vi "NI VeriStand - Get Custom Device Dependencies.vi"(8 "error in (no error)":errorcluster, 11 "Device Ref in":T5 format="%.0x") -> (0 "error out":errorcluster, 2 "Dependencies":T1[](array[typedef]), 3 "Device Ref out":T5 format="%.0x")   [LabVIEW 2020, in "Custom Device Offline API.lvlib"]
uses:
  <vilib>/NI VeriStand/Custom Device Offline API/Custom Device Offline API.lvlib
  <vilib>/NI VeriStand/Custom Device API/Custom Device Item Ref.ctl
  <vilib>/NI VeriStand/Custom Device API/Custom Device File Dependency.ctl
  <vilib>/NI VeriStand/Custom Device API/Path Specification.ctl
  <vilib>/NI VeriStand/Custom Device API/Path Type.ctl
  <vilib>/NI VeriStand/Custom Device API/Custom Device Supported Target.ctl
  NationalInstruments.VeriStand.SystemDefinitionAPI
  <vilib>/NI VeriStand/Custom Device API/Custom Device API.lvlib
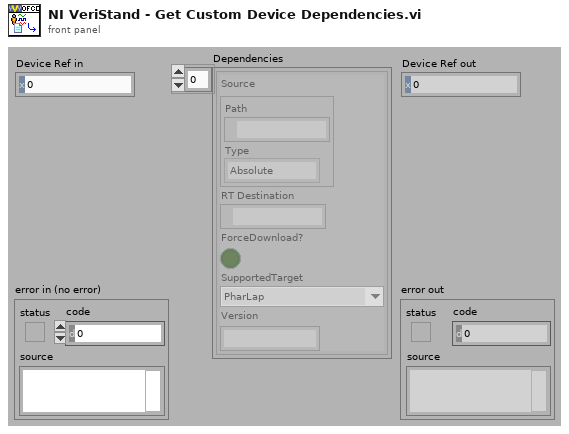
[diagram p1: front panel]
types:
  T1 = typedef "Custom Device API.lvlib/Custom Device File Dependency.ctl" = cluster{"Source":T2, "RT Destination":path, "ForceDownload?":bool, "SupportedTarget":T4, "Version":string}
  T2 = typedef "Custom Device API.lvlib/Path Specification.ctl" = cluster{"Path":path, "Type":T3}
  T3 = typedef "Custom Device API.lvlib/Path Type.ctl" = enum16{"Absolute", "To Base", "To Common Data Dir", "To Application Data Dir"}
  T4 = typedef "Custom Device API.lvlib/Custom Device Supported Target.ctl" = enum16{"All", "PharLap", "VxWorks", "Windows", "Linux_32_ARM", "Linux_x64", "PharLap & Windows", "PharLap & VxWorks", "VxWorks & Windows"}
  T5 = typedef "Custom Device API.lvlib/Custom Device Item Ref.ctl" = u64
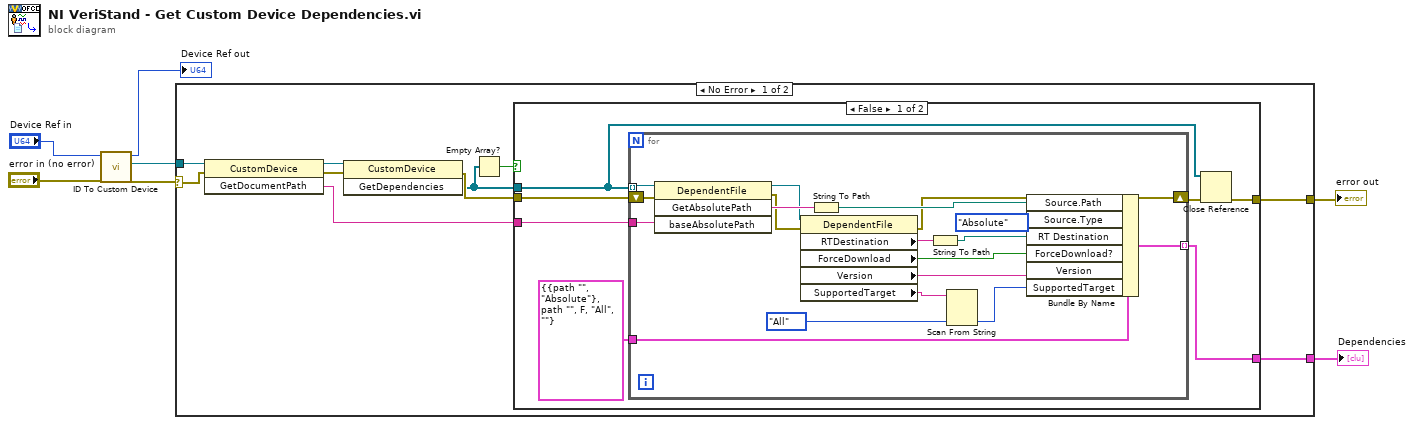
[diagram p0: block diagram]
diagram:
  n1 = call <vilib>:"ID To Custom Device.vi"("error in (no error)"="error in (no error)", "ID in"="Device Ref in") -> ("error out"=w4:errorcluster, "Device"=w3:refnum<k24>, "ID out"=→"Device Ref out":u64)  [unwired: 7 in]
  n2 = case shown="No Error" w4 {
    selector: w4 -> [w16 w44]
    tunnel: w3 -> [w17 _]
    tunnel: [w9 _] -> w2
    tunnel: [w8 w44] -> w1
    frame No Error {
      n3 = invoke class="CustomDevice" method="GetDocumentPath"(reference=w17, error in=w16) -> (reference out=w15:refnum<k24>, error out=w14:errorcluster, "GetDocumentPath"=w12:string)  [unwired: 1 in]
      n4 = invoke class="CustomDevice" method="GetDependencies"(reference=w15, error in=w14) -> (error out=w13:errorcluster, "GetDependencies"=w11:refnum<k24>[])  [unwired: 1 in, 1 out]
      n5 = Empty Array?(array=w11) -> (empty?=w10:bool)
      n6 = case shown="False" w10 {
        tunnel: w13 -> [w23 w43]
        tunnel: w12 -> [w22 _]
        tunnel: w11 -> [w20 _]
        tunnel: [w19 _] -> w9
        tunnel: [w18 w43] -> w8
        frame False {
          n7 = for {
            tunnel: w20 -> [w41] mode=indexing
            tunnel: T1 {"Source"={"Path"=path "", "Type"=enum."Absolute"}, "RT Destination"=path "", "ForceDownload?"=FALSE, "SupportedTarget"=enum."All", "Version"=""} ("Dependency") -> [w42]
            shift-right: [w26] -> w21
            shift-left: w23 -> [w40]
            tunnel: w22 -> [w39]
            tunnel: [w27] -> w19 mode=indexing
            n8 = invoke class="DependentFile" method="GetAbsolutePath"(reference=w41, error in=w40, "baseAbsolutePath"=w39) -> (reference out=w35:refnum<k24>, error out=w34:errorcluster, "GetAbsolutePath"=w38:string)  [unwired: 1 in, 1 out]
            n9 = property class="DependentFile"(reference=w35, error in=w34) -> (error out=w26:errorcluster, "RTDestination"=w33:string, "ForceDownload"=w31:bool, "Version"=w28:string, "SupportedTarget"=w29:string)  [unwired: 1 out]
            n10 = String To Path(string=w38) -> (path=w37:path)
            n11 = String To Path(string=w33) -> (path=w32:path)
            n12 = Scan From String(input string=w29, default 1=Custom_Device_Supported_Target."All" ("SupportedTarget")) -> (output 1=w30:T4)  [unwired: 3 in, 3 out]
            n13 = Bundle By Name(cluster=w42, "Source.Path"=w37, "Source.Type"=Path_Type."Absolute", "RT Destination"=w32, "ForceDownload?"=w31, "Version"=w28, "SupportedTarget"=w30) -> (w27:T1)
          }
          n14 = Close Reference(reference=w20, error in (no error)=w21) -> (error out=w18:errorcluster)
        }
        frame True {
        }
      }
    }
    frame Error {
    }
  }
  "error out" <- w1
  "Dependencies" <- w2
